vi "GetDVR.vi"(8 "error in (no error)":errorcluster, 11 "Mouse":refnum<class "Keyboard.lvclass">) -> (0 "error out":errorcluster, 3 "DVR":refnum<data-value>)   [LabVIEW 2021, in "InputDevice.lvlib" / "Keyboard.lvclass"]
uses:
  Keyboard.lvclass
  data.ctl
  Keyboard.lvclass/Keyboard.ctl
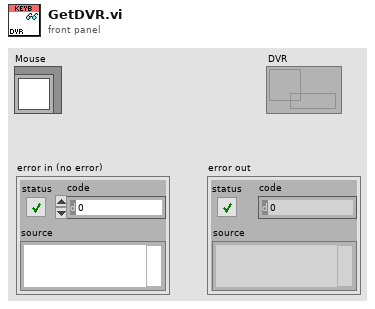
[diagram p1: front panel]
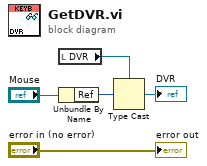
[diagram p0: block diagram]
diagram:
  n1 = local read "DVR"() -> (w4:refnum<data-value>)
  n2 = Unbundle By Name("Mouse") -> ("Ref"=w1:u64)
  n3 = Type Cast(type=w4, x=w1) -> (*(type *) &x=→"DVR":refnum<data-value>)
  "error out" <- "error in (no error)"
